vi "Write Build Specification Version.vi"(8 "error in (no error)":errorcluster, 10 "Build Specification Version":T1, 11 "Task Outputs in":refnum<class "Task Outputs.lvclass">) -> (0 "error out":errorcluster, 3 "Task Outputs out":refnum<class "Task Outputs.lvclass">)   [LabVIEW 2017, in "Message Interface.lvlib" / "Task Outputs.lvclass"]
uses:
  Task Outputs.lvclass
  <vilib>/AppBuilder/AB_API_Simple/Build Specification Version.ctl
  Task Outputs.lvclass/Task Outputs.ctl
  <vilib>/AppBuilder/AB_API_Simple/NI_App_Builder_API.lvlib
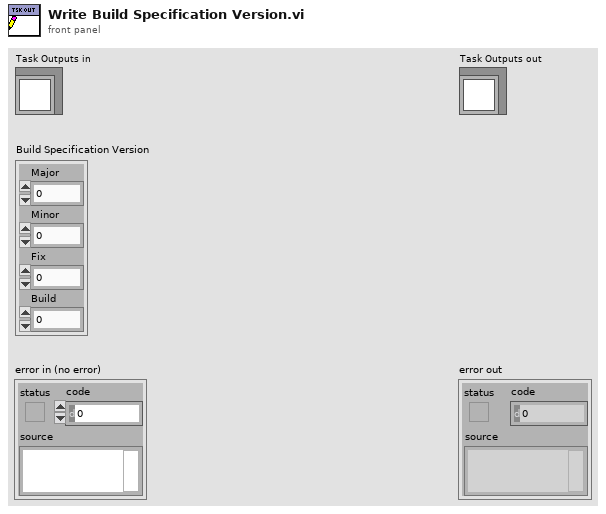
[diagram p1: front panel]
types:
  T1 = typedef "NI_App_Builder_API.lvlib/Build Specification Version.ctl" = cluster{"Major":u16, "Minor":u16, "Fix":u16, "Build":u16}
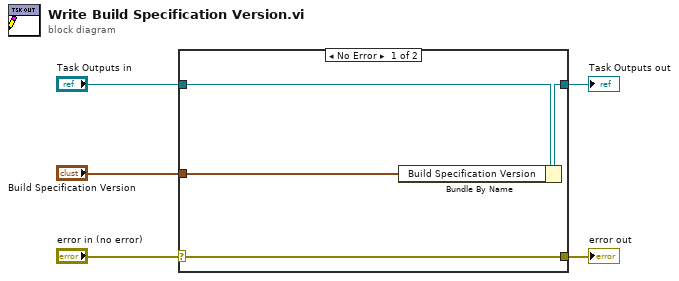
[diagram p0: block diagram]
diagram:
  n1 = case shown="No Error" "error in (no error)" {
    selector: "error in (no error)" -> [w9 w10]
    tunnel: [w9 w10] -> w4
    tunnel: [w7 w11] -> w2
    tunnel: "Task Outputs in" -> [w8 w11]
    tunnel: "Build Specification Version" -> [w6 _]
    frame No Error {
      n2 = Bundle By Name(cluster=w8, "Build Specification Version"=w6) -> (w7:refnum<class "Task Outputs.lvclass">)
    }
    frame Error {
    }
  }
  "error out" <- w4
  "Task Outputs out" <- w2
